vi "Delete State Call.vi"(8 "error in (no error)":errorcluster, 10 "State Call":T1, 11 "JKI SM in":refnum<class "JKI SM.lvclass">) -> (0 "error out":errorcluster, 3 "JKI SM out":refnum<class "JKI SM.lvclass">)   [LabVIEW 2013]
uses:
  JKI State Machine API/source/JKI SM/JKI SM.lvclass
  JKI State Machine API/source/Support/State Call Cluster.ctl
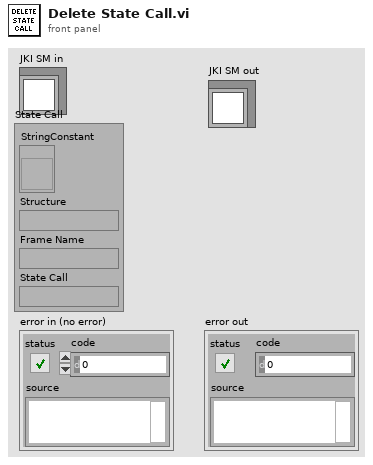
[diagram p1: front panel]
types:
  T1 = typedef "State Call Cluster.ctl" = cluster{"StringConstant":refnum<vi>, "Structure":string, "Frame Name":string, "State Call":string}
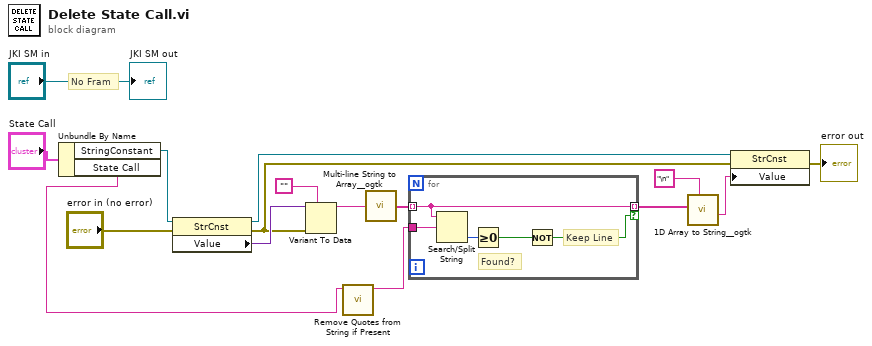
[diagram p0: block diagram]
diagram:
  # "No Fram"
  n1 = Unbundle By Name("State Call") -> ("StringConstant"=w11:refnum<vi>, "State Call"=w1:string)
  n2 = property class="StrCnst"(reference=w11, error in="error in (no error)") -> (reference out=w14:refnum<vi>, error out=w8:errorcluster, "Value"=w10:variant)
  n3 = Variant To Data(error in=w8, type="", Variant=w10) -> (data=w7:string)  [unwired: 1 out]
  n4 = call "Remove Quotes from String if Present.vi"("String"=w1) -> ("String with Quotes Removed"=w5:string)  [unwired: 10 in]
  n5 = call <userlib>:"Multi-line String to Array__ogtk.vi"("string"=w7) -> ("lines"=w6:string[])
  n6 = for {
    tunnel: w6 -> [w18] mode=indexing
    tunnel: w5 -> [w21]
    tunnel: [w18] -> w4 mode=indexing if=w17
    # "Keep Line"
    # "Found?"
    n7 = Search/Split String(string=w18, search string/char (-)=w21) -> (offset of match=w20:i32)  [unwired: 1 in, 2 out]
    n8 = Greater Or Equal To 0?(x=w20) -> (x >= 0?=w19:bool)
    n9 = Not(x=w19) -> (.not. x?=w17:bool)
  }
  n10 = call <userlib>:"1D Array to String__ogtk.vi"("delimiter (Tab)"="\n", "Array of Strings"=w4) -> ("delimited string"=w3:string)  [unwired: 9 in]
  n11 = property class="StrCnst"(reference=w14, error in=w8, "Value"=w3) -> (error out=→"error out":errorcluster)  [unwired: 1 out]
  "JKI SM out" <- "JKI SM in"
